vi "maintenanceTable.vi"() -> ()   [LabVIEW 2020, in "maintenanceLibrary.lvlib"]
uses:
  maintenanceLibrary.lvlib
  <vilib>/measure/mamon.llb/Trigger Detection for 1 Channel.vi
  databaseLibrary.lvlib
  <vilib>/measure/NI_MAPro.lvlib
panel:
  out "status 1":bool
  in  "Close":bool
  out "Table Control":string[][](table)
  # "Maintenance"
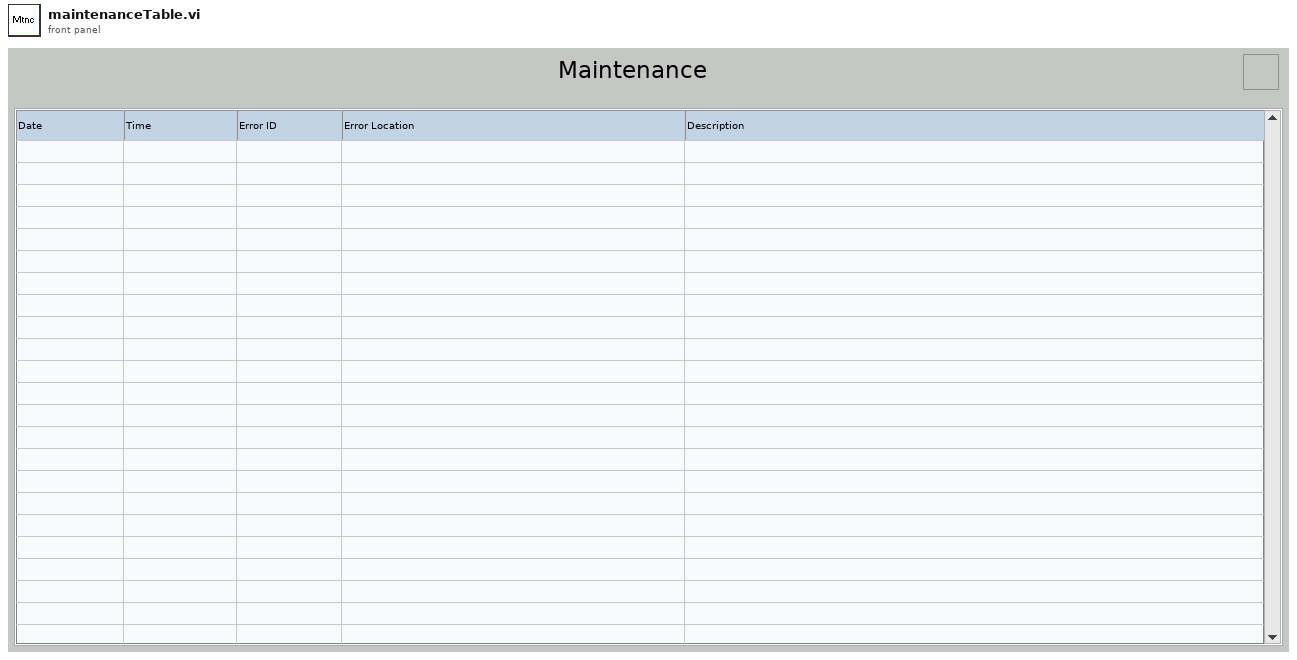
[diagram p1: front panel]
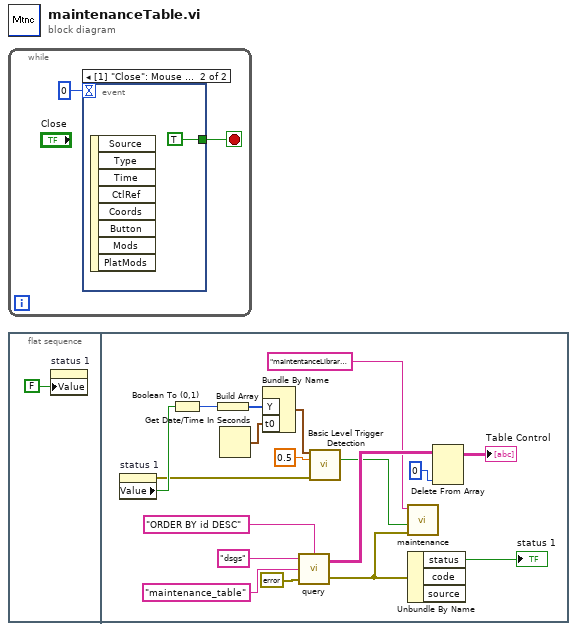
[diagram p0: block diagram]
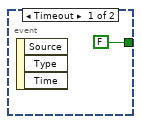
[diagram p2: hidden frame]
diagram:
  n1 = while {
    stop <- w2 stop-if-true
    n2 = event shown="[1] \"Close\": Mouse Down" {
      selector: _ -> [_ _]
      dyn-events: _ -> [_ _]
      timeout: 0 -> [_ _]
      tunnel: [FALSE TRUE] -> w2
      event Timeout {
        n3 = event-data() -> ()  [unwired: 1 in, 3 out]
      }
      event "Close": Mouse Down {
        n4 = event-data() -> ()  [unwired: 1 in, 8 out]
      }
    }
  }
  n5 = flat-sequence {
    frame #0 {
      n6 = property on="status 1" class="Bool (strict)"("Value"=FALSE ("status 1")) -> ()  [unwired: 2 in, 2 out]
    }
    frame #1 {
      n7 = property on="status 1" class="Bool (strict)"() -> (error out=w9:errorcluster, "Value"=w10:bool)  [unwired: 2 in, 1 out]
      n8 = Boolean To (0,1)(Boolean=w10) -> (0, 1=w16:i16)
      n9 = Build Array(w16) -> (w14:i16[])
      n10 = Get Date/Time In Seconds() -> (seconds since 1Jan1904=w15:timestamp)
      n11 = Bundle By Name("Y"=w14, "t0"=w15) -> (w13:waveform(i16))  [unwired: 1 in]
      n12 = call "query.vi"("Condition"="ORDER BY id DESC", "errorIn"=errorcluster {"status"=FALSE, "code"=0, "source"=""} ("Error in"), "Table Name"="maintenance_table", "Connection Name"="dsgs") -> ("errorOut"=w6:errorcluster, "data"=w21:string[][])
      n13 = call-poly <vilib>:"Basic Level Trigger Detection.vi"("signal in"=w13, "level"=0.5, "error in (no error)"=w9) -> ("trigger detected?"=w11:bool)  [unwired: 10 in, 2 out]
      n14 = call "maintenance.vi"("errorIn"=w6, "status"=w11, "errorLocation"="maintentanceLibrary::maintentanceTable.vi") -> ()  [unwired: 8 in, 1 out]
      n15 = Unbundle By Name(w6) -> ("status"=→"status 1":bool)  [unwired: 2 out]
      n16 = Delete From Array(array=w21, index (col)=0 ("disabled index (col)")) -> (array with subset deleted=→"Table Control":string[][])  [unwired: 2 in, 1 out]
    }
  }
